vi "chipKIT UART2 Read.vi"() -> ()   [LabVIEW 2011, in "LabVIEW Interface for ChipKit.lvlib"]
doc: "Read serial data using the secondary UART ont he chipKIT."
uses:
  vi.lib/LabVIEW Interface for ChipKit/LabVIEW Interface for ChipKit.lvlib
  vi.lib/LabVIEW Interface for ChipKit/Private/Type Defs/Chipkit Configuration.ctl
  vi.lib/LabVIEW Interface for ChipKit/Private/Type Defs/Board Type.ctl
panel:
  out "Serial Data":string
  in  "Stop Button":bool
  in  "Buad Rate":u32=9600
  in  "ChipKit Configuration":T1={"COM Port"="COM3", "Board Type"=enum."ChipKit uC32"}
  # "UART2 Read Example\n\nThis example demonstrates how read serial data usring the secondary UART\non the chipKIT\n\nInstructions\n1. Select the COM Port associated with the ChipKit.\n2. Select the Board Type.\n3. Select the Baud Rate for thes secondary UART.\n4. Click the Run Arrow.\n5. Data received on the chipKITs secondary UART is displayed in the Serial Data string control."
  # "chipKIT Settings"
  # "Channel Settings"
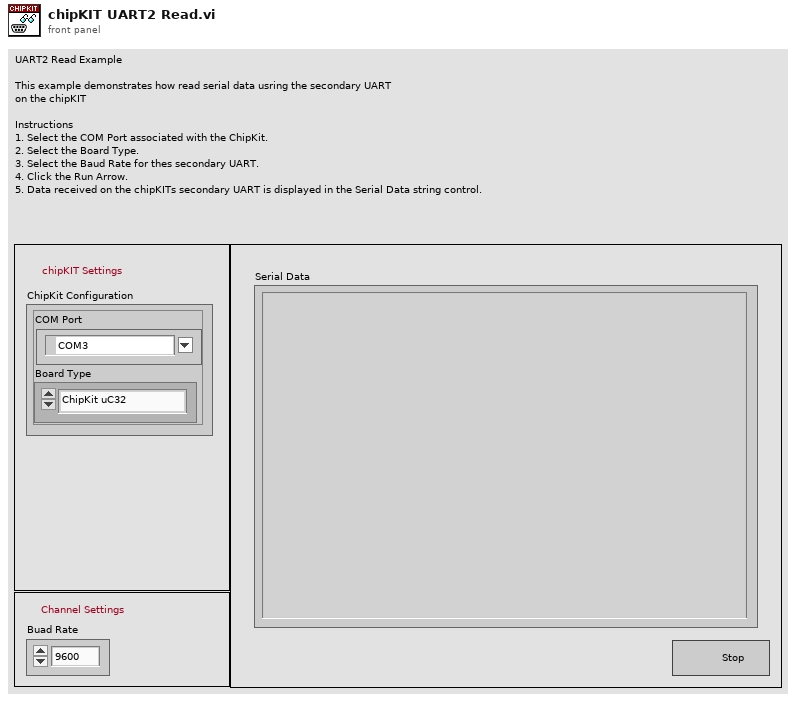
[diagram p1: front panel]
types:
  T1 = typedef "LabVIEW Interface for ChipKit.lvlib/Chipkit Configuration.ctl" = cluster{"COM Port":refnum<visa-resource-name>, "Board Type":T2}
  T2 = typedef "LabVIEW Interface for ChipKit.lvlib/Board Type.ctl" = enum16{"ChipKit uC32", "ChipKit Uno32", "ChipKit Max32"}
  T3 = typedef "LabVIEW Interface for ChipKit.lvlib/Chipkit Resource.ctl" = cluster{"COM Port":refnum<visa-resource-name>, "Board Type":T2, "Connection Type":T4, "Baud Rate (115200)":u32, "Bytes Per Packet (15)":u32, "DI Port Num Pins":i32, "DO Port Num Pins":i32}
  T4 = typedef "LabVIEW Interface for ChipKit.lvlib/Connection Type.ctl" = enum8{"USB / Serial", "XBEE", "BlueSmirf (Bluetooth)"}
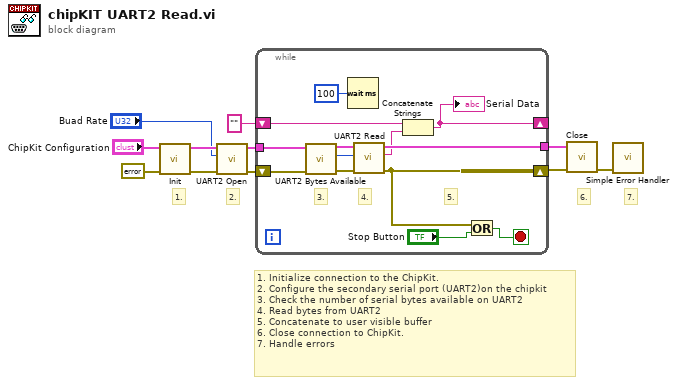
[diagram p0: block diagram]
diagram:
  # "1. Initialize connection to the ChipKit.\n2. Configure the secondary serial port (UART2)on the chipkit\n3. Check the number of serial bytes available on UART2\n4. Read bytes from UART2\n5. Concatenate to user visible buffer\n6. Close connection to ChipKit.\n7. Handle errors"
  # "7."
  # "6."
  # "2."
  # "1."
  n1 = call "Init.vi"("Error In"=errorcluster {"status"=FALSE, "code"=0, "source"=""}, "ChipKit Configuration"="ChipKit Configuration") -> ("Error Out"=w7:errorcluster, "ChipKit Configuration"=w11:T3)  [unwired: 8 in]
  n2 = call "UART2 Open.vi"("Error In"=w7, "Buad Rate"="Buad Rate", "ChipKit Resource"=w11) -> ("Error Out"=w8:errorcluster, "ChipKit Resource"=w10:T3)  [unwired: 7 in]
  n3 = while {
    tunnel: w10 -> [w19]
    shift-right: [w15] -> w9
    shift-left: w8 -> [w21]
    tunnel: [w16] -> w3
    shift-right: [w12] -> _
    shift-left: "" -> [w14]
    stop <- w23 stop-if-true
    # "5."
    # "4."
    # "3."
    n4 = call "UART2 Bytes Available.vi"("Error In"=w21, "ChipKit Resource"=w19) -> ("Error Out"=w20:errorcluster, "Bytes Available"=w17:u8, "ChipKit Resource"=w18:T3)  [unwired: 7 in]
    n5 = Wait (ms)(milliseconds to wait=u32 100) -> ()  [unwired: 1 out]
    n6 = call "UART2 Read.vi"("Error In"=w20, "Bytes To Read"=w17, "ChipKit Resource"=w18) -> ("Error Out"=w15:errorcluster, "Data"=w13:string, "ChipKit Resource"=w16:T3)  [unwired: 6 in]
    n7 = Concatenate Strings(w14, w13) -> (w12:string)
    "Serial Data" <- w12
    n8 = Or(x=w15, y="Stop Button") -> (x .or. y?=w23:bool)
  }
  n9 = call "Close.vi"("Error In"=w9, "ChipKit Configuration"=w3) -> ("Error Out"=w1:errorcluster)  [unwired: 9 in]
  n10 = call <vilib>:"Simple Error Handler.vi"("error in (no error)"=w1) -> ()  [unwired: 4 in, 5 out]
